vi "Get Policy Version Details.vi"(8 "error in (no error)":errorcluster, 9 "Version":i32, 10 "Name":string, 11 "IoT Session in":refnum<class "IoT Session.lvclass">) -> (0 "error out":errorcluster, 1 "Default Version":bool, 2 "Details":T1, 3 "IoT Session out":refnum<class "IoT Session.lvclass">)   [LabVIEW 2015, in "NI_AWS_IoT.lvlib" / "IoT Session.lvclass"]
uses:
  IoT Session.lvclass
  Policy.ctl
  Core/HTTP Request/Request Options.ctl
  Core/HTTP Request/Name Value Pair.ctl
  Core/HTTP Request/Region handling.ctl
  Core/HTTP Request/URL formatting.ctl
  Core/HTTP Request/HTTP Request.lvclass
  JSON Parsing/NI_JSON Parsing.lvlib
  NI_AWS_IoT.lvlib
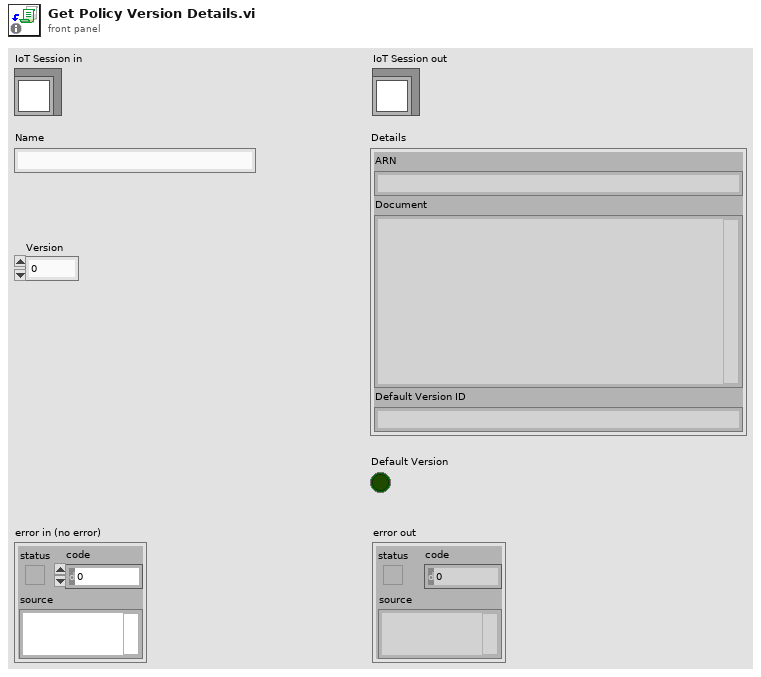
[diagram p1: front panel]
types:
  T1 = typedef "NI_AWS_IoT.lvlib/Policy.ctl" = cluster{"ARN":string, "Document":string, "Default Version ID":string}
  T2 = typedef "NI_AWS_Core.lvlib/HTTP Request.lvclass/Name Value Pair.ctl" = cluster{"name":string, "value":string}
  T3 = typedef "NI_AWS_Core.lvlib/HTTP Request.lvclass/Request Options.ctl" = cluster{"request headers":T2[], "request parameters":T2[], "request body":string, "region handling":T4, "URL formatting":T5}
  T4 = typedef "NI_AWS_Core.lvlib/HTTP Request.lvclass/Region handling.ctl" = enum16{"use region everywhere", "use region (authentication only)", "use region (URL only)", "ignore region everwhere"}
  T5 = typedef "NI_AWS_Core.lvlib/HTTP Request.lvclass/URL formatting.ctl" = enum16{"region-", "region."}
  T6 = typedef "NI_AWS_Core.lvlib/HTTP Request.lvclass/Response.ctl" = cluster{"Headers":string, "Body":string}
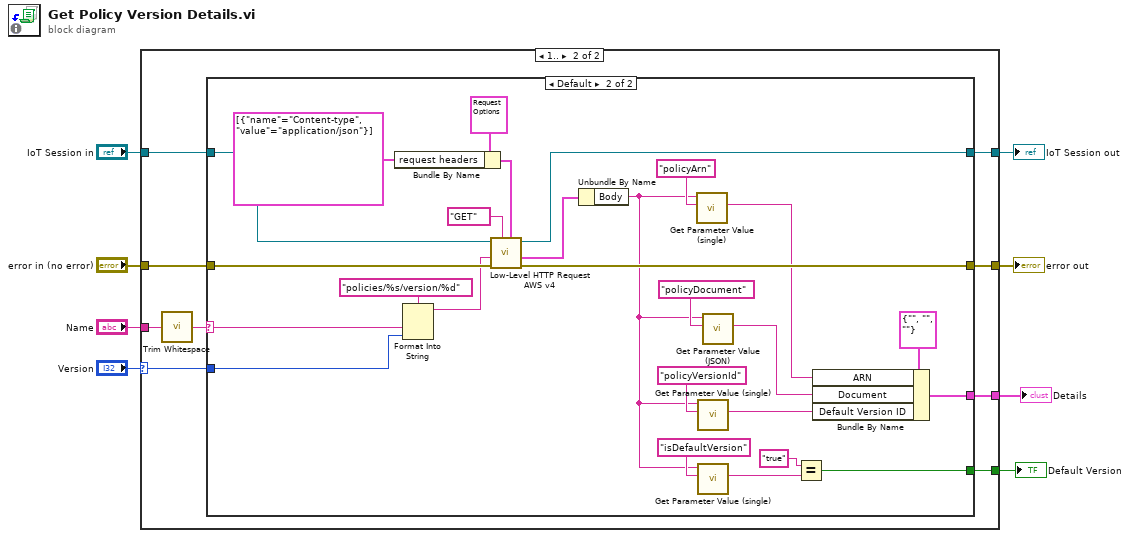
[diagram p0: block diagram]
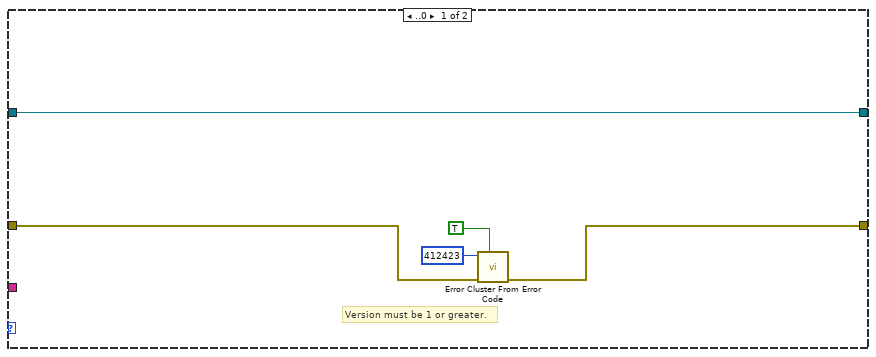
[diagram p2: hidden frame]
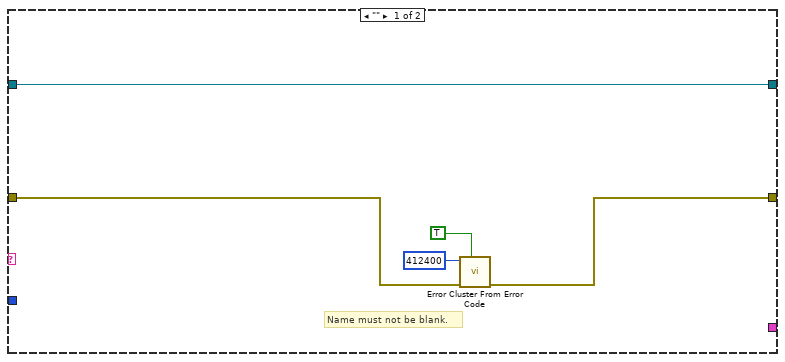
[diagram p3: hidden frame]
diagram:
  n1 = case shown="1.." "Version" {
    selector: "Version" -> [_ w16]
    tunnel: "error in (no error)" -> [w10 w22]
    tunnel: [w9 w21] -> w7
    tunnel: [w13 w20] -> w6
    tunnel: "IoT Session in" -> [w13 w19]
    tunnel: [_ w18] -> w4
    tunnel: "Name" -> [_ w17]
    tunnel: [_ w14] -> w1
    frame ..0 {
      # "Version must be 1 or greater."
      n2 = call <vilib>:"Error Cluster From Error Code.vi"("show call chain? (False)"=TRUE, "error in (no error)"=w10, "error code (0)"=412423) -> ("error out"=w9:errorcluster)  [unwired: 6 in]
    }
    frame 1.. {
      n3 = call <vilib>:"Trim Whitespace.vi"("string"=w17) -> ("trimmed string"=w15:string)  [unwired: 1 in]
      n4 = case shown="Default" w15 {
        selector: w15 -> [_ w34]
        tunnel: w22 -> [w25 w53]
        tunnel: [w24 w52] -> w21
        tunnel: [w23 w51] -> w20
        tunnel: w19 -> [w23 w50]
        tunnel: [_ w42] -> w18
        tunnel: w16 -> [_ w33]
        tunnel: [_ w28] -> w14
        frame "" {
          # "Name must not be blank."
          n5 = call <vilib>:"Error Cluster From Error Code.vi"("show call chain? (False)"=TRUE, "error in (no error)"=w25, "error code (0)"=412400) -> ("error out"=w24:errorcluster)  [unwired: 6 in]
        }
        frame Default {
          n6 = Bundle By Name(cluster=T3 {"request headers"=[], "request parameters"=[], "request body"="", "region handling"=enum."use region everywhere", "URL formatting"=enum."region."} ("Request Options"), "request headers"=T2[] [{"name"="Content-type", "value"="application/json"}]) -> (w47:T3)
          n7 = Format Into String(format string="policies/%s/version/%d" ("string"), w34, w33) -> (resulting string=w36:string)  [unwired: 2 in, 1 out]
          n8 = call "Low-Level HTTP Request AWS v4.vi"("Request Options"=w47, "HTTP-Verb"="GET", "error in (no error)"=w53, "URL Suffix"=w36, "AWS Core in"=w50) -> ("error out"=w52:errorcluster, "Response"=w45:T6, "AWS Core out"=w51:refnum<class "IoT Session.lvclass">)  [unwired: 3 in, 1 out]
          n9 = Unbundle By Name(w45) -> ("Body"=w31:string)
          n10 = call "Get Parameter Value (single).vi"("Parameter Name"="policyArn", "JSON"=w31) -> ("Parameter Value"=w41:string)  [unwired: 6 in, 3 out]
          n11 = call "Get Parameter Value (single).vi"("Parameter Name"="policyVersionId", "JSON"=w31) -> ("Parameter Value"=w39:string)  [unwired: 6 in, 3 out]
          n12 = call "Get Parameter Value (single).vi"("Parameter Name"="isDefaultVersion", "JSON"=w31) -> ("Parameter Value"=w30:string)  [unwired: 6 in, 3 out]
          n13 = call "Get Parameter Value (JSON).vi"("Parameter Name"="policyDocument", "JSON"=w31) -> ("Parameter Value"=w37:string)  [unwired: 6 in, 3 out]
          n14 = Equal?(x="true", y=w30) -> (x = y?=w28:bool)
          n15 = Bundle By Name(cluster=T1 {"ARN"="", "Document"="", "Default Version ID"=""} ("Details"), "ARN"=w41, "Document"=w37, "Default Version ID"=w39) -> (w42:T1)
        }
      }
    }
  }
  "error out" <- w7
  "IoT Session out" <- w6
  "Details" <- w4
  "Default Version" <- w1
